vi "Global_CMD_ACT_Data In.vi"() -> ()   [LabVIEW 2020, in "Swerve AM_ACT.lvlib"]
uses:
  Swerve AM_ACT.lvlib
  Cluster_CMD_ACT_Data.ctl
  ENUM_CMD_Mode Select.ctl
  Shared Code/TypeDefs/Cluster_CMD_Direction Data.ctl
  Shared Code/TypeDefs/Cluster_Module Velocity-Direction-Rotations.ctl
  Shared Code/TypeDefs/Level_Velocity plus-minus 1.ctl
  Shared Code/TypeDefs/Dial_Compase heading unit circle CCW positive.ctl
  Shared Code/TypeDefs/Cluster_X-Y.ctl
panel:
  in  "CMD_ACT_Tempplate Data":T1 {"Target Auto Angle" scale format="%.3f"; "Direction"."Rotate(Yaw) CCW 1 CW -1" scale=1.0..-1.0; "Direction"."Traverse"."Angle" scale format="%.3f"; "Direction"."Traverse"."Velocity" scale=-1.0..1.0 scale format="%.1f"}
  # "The Names of the Data items in the Global Variable MUST describe who the Single Writer is\nFor Command Globals the Commander(CMD) represents Teleop or Autonomous or other command loop.\nThe naming convention for a Command Actuator Global is:   \n\nCMD_ACT_SubSystem_Data Name\n\nExample:\nCMD_ACT_Drive_Data\nCMD_ACT_Hopper_Eject Ball"
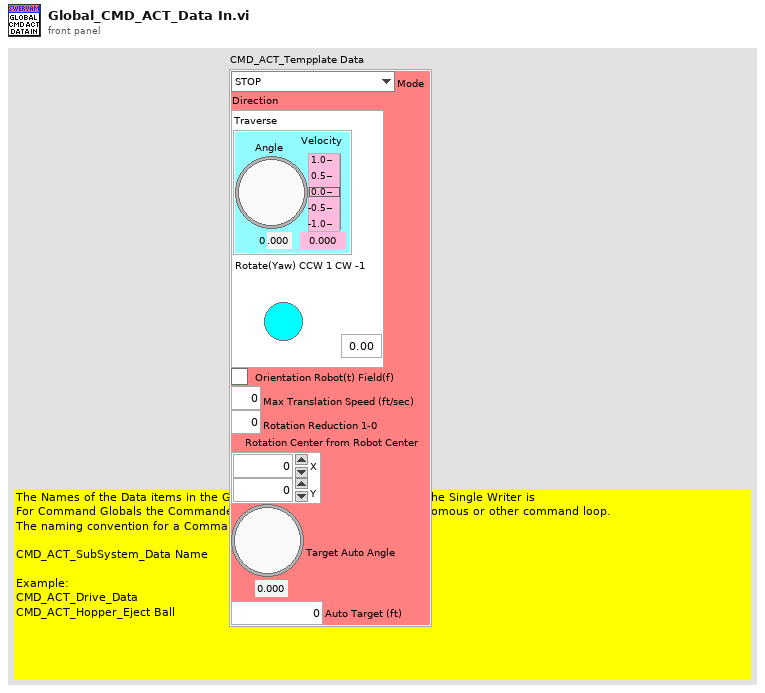
[diagram p1: front panel]
types:
  T1 = typedef "Swerve AM_ACT.lvlib/Cluster_CMD_ACT_Data.ctl" = cluster{"Mode":T2, "Direction":T3, "Orientation Robot(t) Field(f)":bool, "Max Translation Speed (ft/sec)":dbl, "Rotation Reduction 1-0":dbl, "Rotation Center from Robot Center":T7, "Target Auto Angle":T6, "Auto Target (ft)":dbl}
  T2 = typedef "Swerve AM_ACT.lvlib/ENUM_CMD_Mode Select.ctl" = enum16{"STOP", "Move", "Turret Manual", "Trans Manual Angle Auto", "Turret Auto Angle"}
  T3 = typedef "Cluster_CMD_Direction Data.ctl" = cluster{"Traverse":T4, "Rotate(Yaw) CCW 1 CW -1":dbl}
  T4 = typedef "Cluster_Module Velocity-Direction-Rotations.ctl" = cluster{"Velocity":T5, "Angle":T6, "Rotations Count":dbl}
  T5 = typedef "Level_Velocity plus-minus 1.ctl" = dbl
  T6 = typedef "Dial_Compase heading unit circle CCW positive.ctl" = dbl
  T7 = typedef "Cluster_X-Y.ctl" = cluster{"X":dbl, "Y":dbl}
diagram:
